vi "Robot Global Data.vi"() -> ()   [LabVIEW 2013]
doc: "This global VI can contain as many global variables as you need. Place a control on the panel, give it a good name. To read or write to it from a VI, drag the icon to the diagram of that VI. You can also drag from the project. Click on the node to change which global you access. You shouldn't have multiple locations writing to a global or it will cause a race-condition."
uses:
  <vilib>/Rock Robotics/WPI/Camera/WPI_CameraImageSize.ctl
  <vilib>/Rock Robotics/WPI/DriverStation/WPI_DriverStationRobotMode2.ctl
  Encoder Values.ctl
  <vilib>/Rock Robotics/WPI/Joystick/WPI_JoystickButtonState.ctl
  Autonomous Commands.ctl
  Shoot Location.ctl
  UDP Dashboard Packet.ctl
  Autonomous Setpoints.ctl
  Auto Shift Settings.ctl
  Shoot Profile.ctl
  Halo Drive.ctl
  Auto Speed Constants.ctl
  Autonomous Center Line Setpoints.ctl
panel:
  out "UDP Packet":T1={"Feed Angle"=20.0, "Neutral Angle"=25.8, "Autonomous Setpoints"={"Shoot Angle 1"=15.4, "Initial Delay"=0.0, "Disc Count 1"=3.0, "Shoot Time 1"=8000.0, "Distance 1"=6.5, "Two Disc Distance 1"=4.0, "Distance 2"=10.5, "Two Disc Distance 2"=6.0, "Distance 3"=-10.0, "Two Disc Distance 3"=0.0, "Shoot Angle 3"=23.0, "Disc Count 3"=5.0, "Shoot Time 3"=15000.0, "Distance 4"=0.0, "Two Disc Distance 4"=0.0, "Low Gear"=TRUE, "Shoot 1 Post Delay"=250.0}, "Auto Shift"={"Enabled"=FALSE, "Upshift Speed"=20.0, "Downshift Speed"=20.0, "Upshift Throttle"=0.6000000000000001, "Turn Power Diff"=0.7, "Motor Limit"=400.0, "Encoder Limit"=100.0}, "Elevator Angle Offset"=0.0, "Potentiometer Angle"={"Pot M"=42.09, "Pot B"=-65.397}, "Shoot Setpoints"={"Vision"={"Pre RPM"=3500.0, "Main RPM"=4000.0, "Angle"=16.4}, "Back Corner"={"Pre RPM"=3500.0, "Main RPM"=4000.0, "Angle"=16.3}, "Front"={"Pre RPM"=3500.0, "Main RPM"=4000.0, "Angle"=23.5}, "Front Corner"={"Pre RPM"=3500.0, "Main RPM"=4000.0, "Angle"=21.8}, "Half Court"={"Pre RPM"=3500.0, "Main RPM"=4000.0, "Angle"=16.4}, "Full Court"={"Pre RPM"=4500.0, "Main RPM"=5000.0, "Angle"=16.0}, "Pyramid"={"Pre RPM"=2800.0, "Main RPM"=3300.0, "Angle"=28.0}}, "Halo Drive"={"Gains"={"Quickturn_Sens_Low"=1.2, "Quickturn_Sens_High"=1.0, "Speedturn_Sens_Low"=1.5, "Speedturn_Sens_High"=1.7}, "QuickTurn Const"=0.25, "Loading Throttle Limit"=0.5}, "Auto Speed Constants"={"Slowing Distance"=0.5, "High Speed"=0.8999999999999999, "Rampup Time"=500.0, "Low Speed"=0.5, "High Speed (Reverse)"=0.8999999999999999}, "Shooting Delays"={"Unjam On"=100.0, "Unjam Off"=100.0, "Flipper On"=300.0, "Flipper Off"=200.0, "Hopper Up"=100.0}, "Left Roller Pwr"=0.8, "Right Roller Pwr"=0.8, "Elevator PID Gains"={"proportional gain (Kc)"=0.2, "integral time (Ti, min)"=0.0, "derivative time (Td, min)"=0.002}, "Elevator PID Output Range"={"output high"=1.0, "output low"=-1.0}, "Elevator Angle Tolerance"=0.1, "Toggle Ears Delay"=500.0, "Toggle Ears Distance"=2.0, "Unjam Servo Angle"=93.0, "Auton Steer PID gains"={"proportional gain (Kc)"=0.007, "integral time (Ti, min)"=0.0, "derivative time (Td, min)"=0.0}, "Auton Steer output range"={"output high"=1.0, "output low"=-1.0}, "Auto Reverse Speed"=0.2, "Auto Stop Throttle"=0.0, "Auto Stop Duration"=0.0, "Spin output range"={"output high"=1.0, "output low"=-1.0}, "Spin PID gains"={"proportional gain (Kc)"=0.4, "integral time (Ti, min)"=0.0, "derivative time (Td, min)"=0.0}, "Auto-Center Line"={"Arc Turn x-axis"=0.0, "Arc Turn y-axis"=0.8999999999999999, "Arc Turn Distance"=-11.0, "Distance 1"=11.0, "Two Disc Distance 1"=0.0, "Distance 2"=-2.0, "Two Disc Distance 2"=0.0, "Spin Angle"=-70.0, "Spin Angle tolerance"=5.0, "Spin y-axis"=0.0, "Spin Distance"=0.0, "Center Line Enabled"=FALSE, "Distance 3"=12.0, "Two Disc Distance 3"=0.0, "Spin Angle 2"=85.0, "Spin Angle tolerance 2"=15.0, "Spin y-axis 2"=0.0, "Spin Distance 2"=0.0, "Shoot Angle 1"=14.6, "Disc Count 1"=3.0, "Shoot Time 1"=8000.0, "Shoot Angle 3"=18.4, "Disc Count 3"=5.0, "Shoot Time 3"=15000.0, "Low Gear"=TRUE}, "Auton Distance PID gains Low Gear"={"proportional gain (Kc)"=0.9999999999999999, "integral time (Ti, min)"=0.007, "derivative time (Td, min)"=0.0}, "Auton Distance output range"={"output high"=0.9, "output low"=-0.9}, "Auton Distance Threshold"=0.25, "Auton Velocity Cutoff"=1.5, "Auton Distance output range Center Line"={"output high"=1.0, "output low"=-1.0}, "Auton Distance PID gains High Gear"={"proportional gain (Kc)"=0.9999999999999999, "integral time (Ti, min)"=0.007, "derivative time (Td, min)"=0.0}} {"Auton Distance PID gains High Gear"."derivative time (Td, min)" format="%.3f"; "Auton Distance PID gains High Gear"."integral time (Ti, min)" format="%.3f"; "Auton Distance PID gains High Gear"."proportional gain (Kc)" format="%.3f"; "Auton Distance PID gains Low Gear"."derivative time (Td, min)" format="%.3f"; "Auton Distance PID gains Low Gear"."integral time (Ti, min)" format="%.3f"; "Auton Distance PID gains Low Gear"."proportional gain (Kc)" format="%.3f"; "Spin PID gains"."derivative time (Td, min)" format="%.3f"; "Spin PID gains"."integral time (Ti, min)" format="%.3f"; "Spin PID gains"."proportional gain (Kc)" format="%.3f"; "Spin output range"."output low" format="%.2f"; "Spin output range"."output high" format="%.2f"; "Auton Steer PID gains"."derivative time (Td, min)" format="%.3f"; "Auton Steer PID gains"."integral time (Ti, min)" format="%.3f"; "Auton Steer PID gains"."proportional gain (Kc)" format="%.3f"}
  in  "Shoot Location":T8
  in  "Auton Commands":T9
  in  "Azimuth Low Gear":bool
  in  "Azimuth Ready":bool
  out "Gryo Angle":dbl
  out "Drive Controls":T10
  in  "Shooter Mode":T11(ring)=enum."Neutral Angle"
  out "Disc Count":dbl
  in  "RPM Min Percentage":dbl
  in  "RPM Max Percentage":dbl
  in  "Bangbang Smooth":dbl
  in  "Target Pre RPM":dbl
  in  "Elevator Target Angle":dbl
  out "IR Sensors":T12
  out "Joysticks":T14
  in  "Drive Limit":bool
  in  "Disc Mode":enum16{"Drive", "Load", "Shoot", "Feed"}(ring)
  in  "Shooter Manual Power":bool
  out "Encoder Values":T15
  in  "Low Gear":bool
  in  "Shooter Active":bool
  in  "Target Main RPM":dbl
  in  "Robot Mode":T16
  in  "LED toggle rate (ms)":u32=20
  in  "image size":T17=enum."320x240"
  in  "Enable Vision":bool
  # "\"Target\" is one of the choices in UDP packet,\nbased on the driver's \"shoot location\""
  # "Low level, controlled by\nShooter Mode in auto loop"
  # "High level, auto controlled state"
  # "Pre RPM"
  # "Main RPM"
  # "Angle"
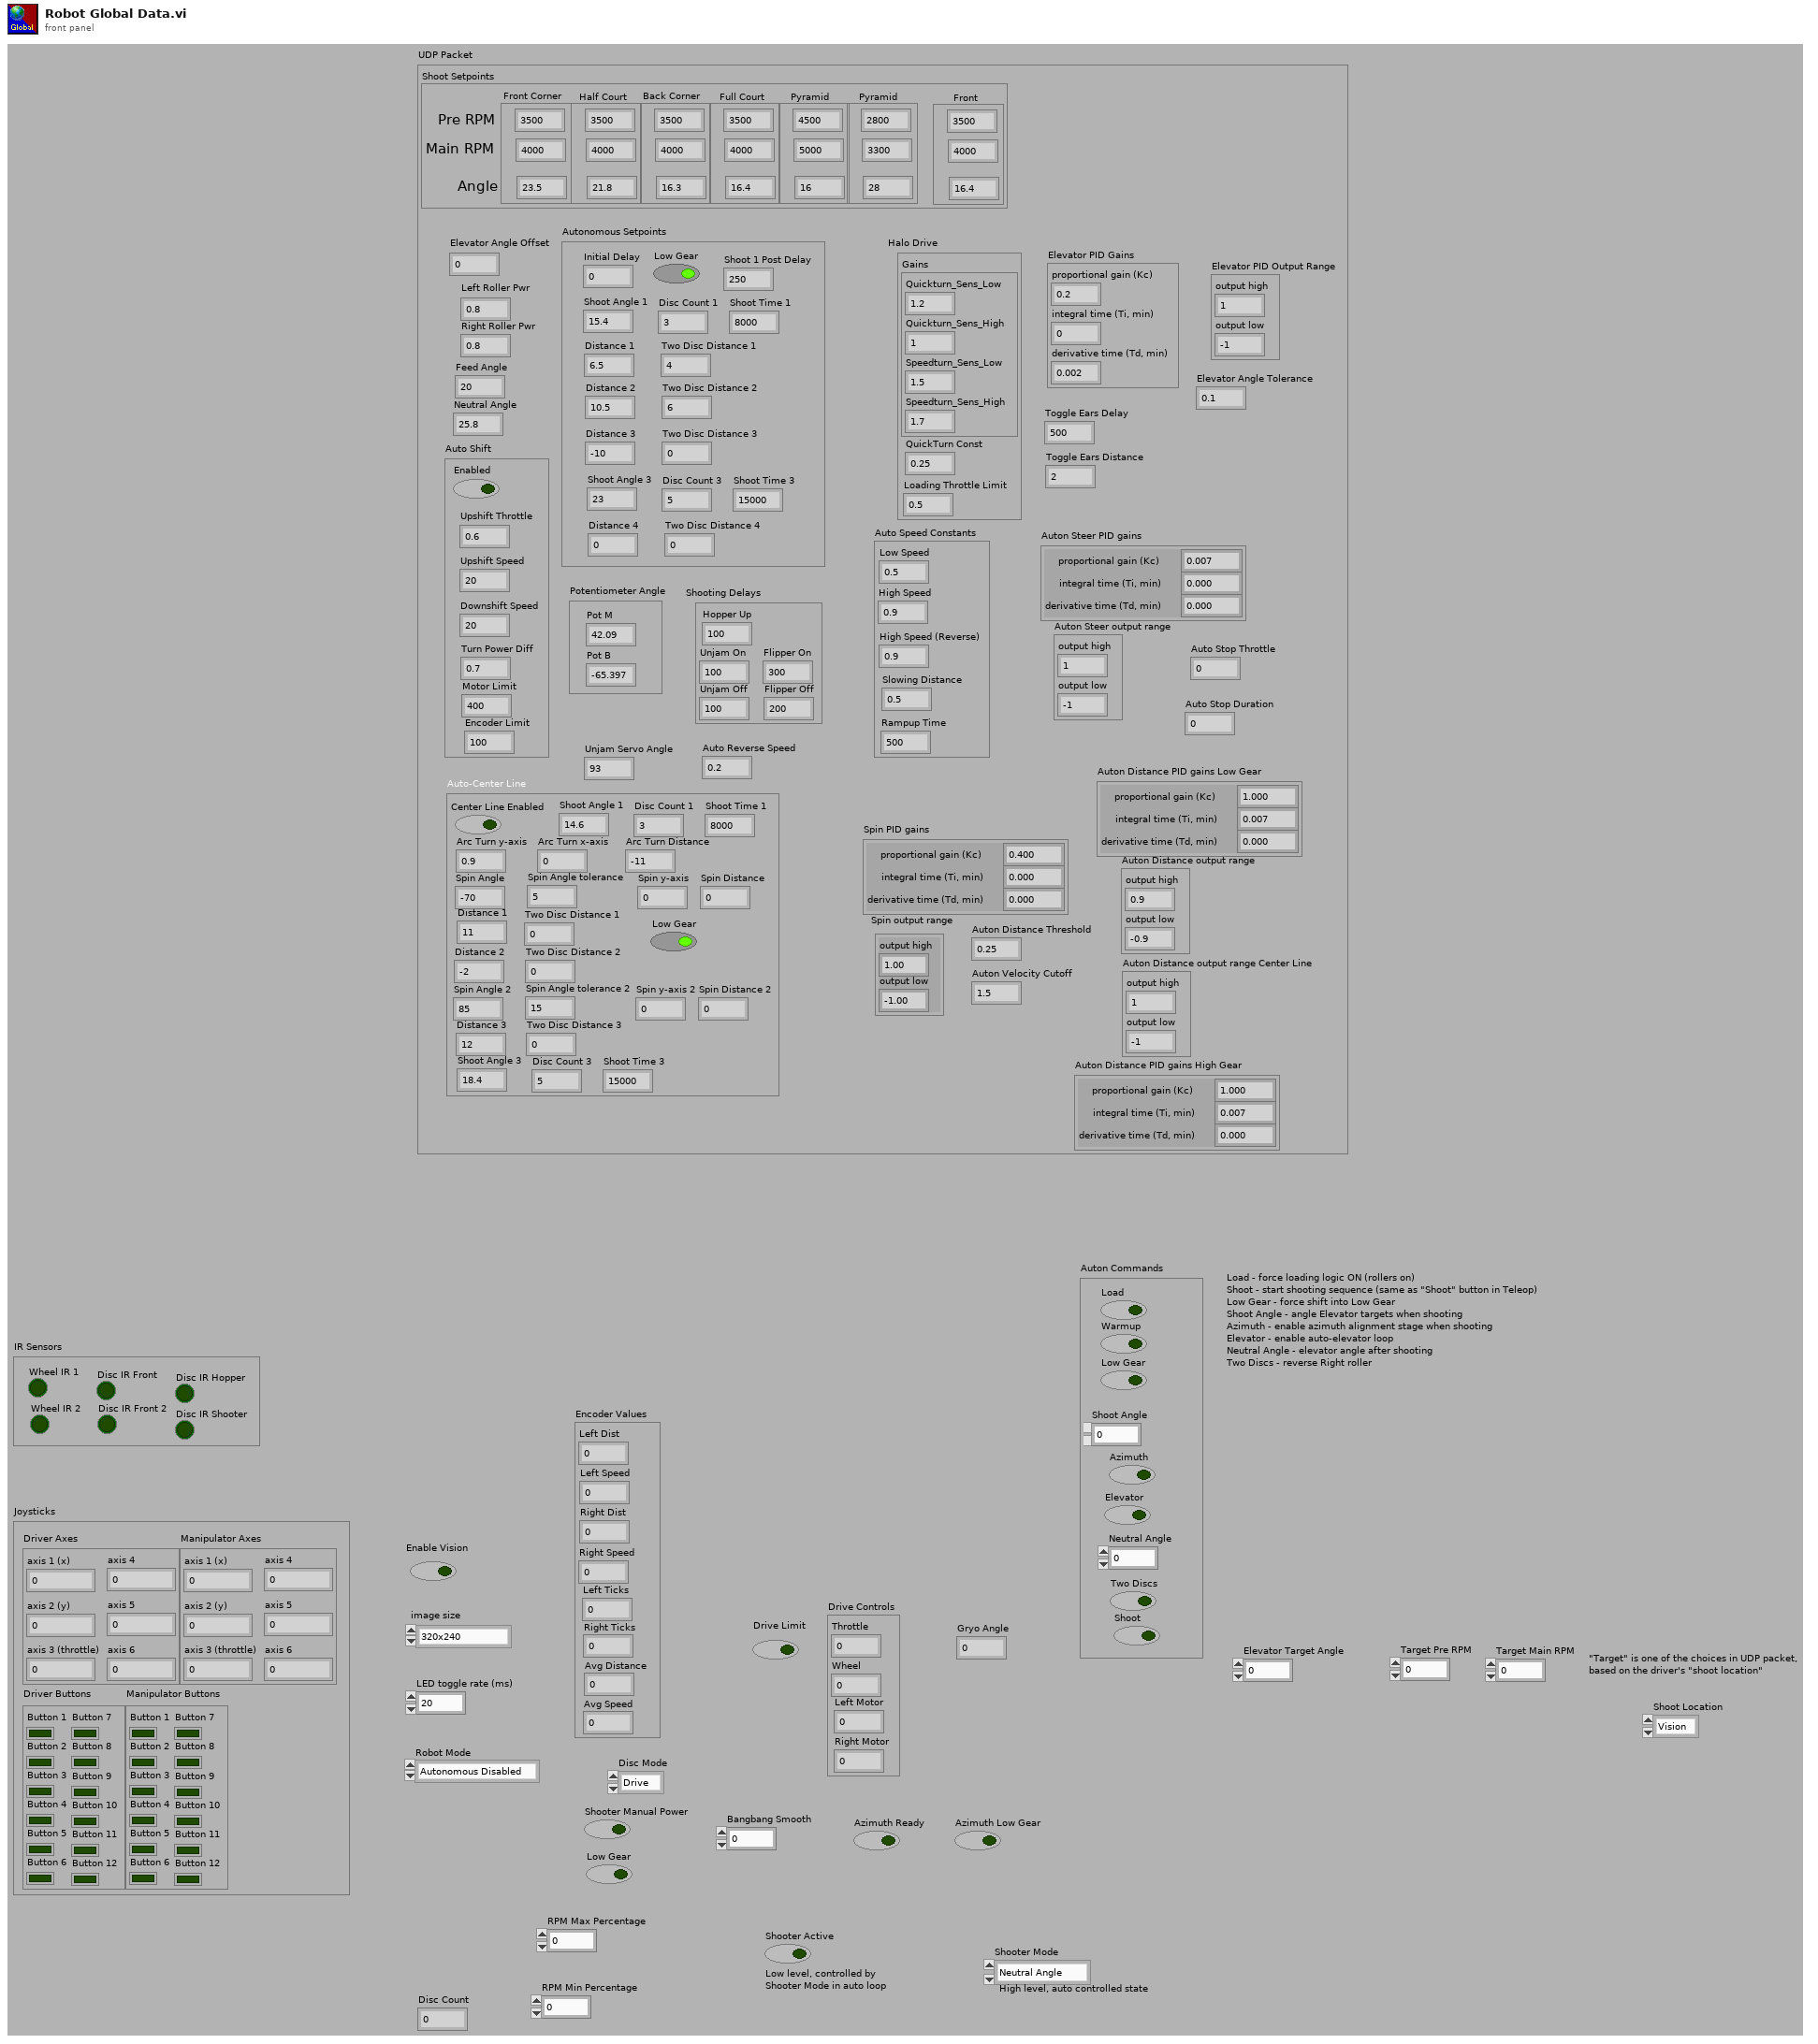
[diagram p1: front panel]
types:
  T1 = typedef "UDP Dashboard Packet.ctl" = cluster{"Feed Angle":dbl, "Neutral Angle":dbl, "Autonomous Setpoints":T2, "Auto Shift":T3, "Elevator Angle Offset":dbl, "Potentiometer Angle":cluster{"Pot M":dbl, "Pot B":dbl}, "Shoot Setpoints":cluster{"Vision":T4, "Back Corner":T4, "Front":T4, "Front Corner":T4, "Half Court":T4, "Full Court":T4, "Pyramid":T4}, "Halo Drive":T5, "Auto Speed Constants":T6, "Shooting Delays":cluster{"Unjam On":dbl, "Unjam Off":dbl, "Flipper On":dbl, "Flipper Off":dbl, "Hopper Up":dbl}, "Left Roller Pwr":dbl, "Right Roller Pwr":dbl, "Elevator PID Gains":cluster{"proportional gain (Kc)":dbl, "integral time (Ti, min)":dbl, "derivative time (Td, min)":dbl}, "Elevator PID Output Range":cluster{"output high":dbl, "output low":dbl}, "Elevator Angle Tolerance":dbl, "Toggle Ears Delay":dbl, "Toggle Ears Distance":dbl, "Unjam Servo Angle":dbl, "Auton Steer PID gains":cluster{"proportional gain (Kc)":dbl, "integral time (Ti, min)":dbl, "derivative time (Td, min)":dbl}, "Auton Steer output range":cluster{"output high":dbl, "output low":dbl}, "Auto Reverse Speed":dbl, "Auto Stop Throttle":dbl, "Auto Stop Duration":dbl, "Spin output range":cluster{"output high":dbl, "output low":dbl}, "Spin PID gains":cluster{"proportional gain (Kc)":dbl, "integral time (Ti, min)":dbl, "derivative time (Td, min)":dbl}, "Auto-Center Line":T7, "Auton Distance PID gains Low Gear":cluster{"proportional gain (Kc)":dbl, "integral time (Ti, min)":dbl, "derivative time (Td, min)":dbl}, "Auton Distance output range":cluster{"output high":dbl, "output low":dbl}, "Auton Distance Threshold":dbl, "Auton Velocity Cutoff":dbl, "Auton Distance output range Center Line":cluster{"output high":dbl, "output low":dbl}, "Auton Distance PID gains High Gear":cluster{"proportional gain (Kc)":dbl, "integral time (Ti, min)":dbl, "derivative time (Td, min)":dbl}}
  T2 = typedef "Autonomous Setpoints.ctl" = cluster{"Shoot Angle 1":dbl, "Initial Delay":dbl, "Disc Count 1":dbl, "Shoot Time 1":dbl, "Distance 1":dbl, "Two Disc Distance 1":dbl, "Distance 2":dbl, "Two Disc Distance 2":dbl, "Distance 3":dbl, "Two Disc Distance 3":dbl, "Shoot Angle 3":dbl, "Disc Count 3":dbl, "Shoot Time 3":dbl, "Distance 4":dbl, "Two Disc Distance 4":dbl, "Low Gear":bool, "Shoot 1 Post Delay":dbl}
  T3 = typedef "Auto Shift Settings.ctl" = cluster{"Enabled":bool, "Upshift Speed":dbl, "Downshift Speed":dbl, "Upshift Throttle":dbl, "Turn Power Diff":dbl, "Motor Limit":dbl, "Encoder Limit":dbl}
  T4 = typedef "Shoot Profile.ctl" = cluster{"Pre RPM":dbl, "Main RPM":dbl, "Angle":dbl}
  T5 = typedef "Halo Drive.ctl" = cluster{"Gains":cluster{"Quickturn_Sens_Low":dbl, "Quickturn_Sens_High":dbl, "Speedturn_Sens_Low":dbl, "Speedturn_Sens_High":dbl}, "QuickTurn Const":dbl, "Loading Throttle Limit":dbl}
  T6 = typedef "Auto Speed Constants.ctl" = cluster{"Slowing Distance":dbl, "High Speed":dbl, "Rampup Time":dbl, "Low Speed":dbl, "High Speed (Reverse)":dbl}
  T7 = typedef "Autonomous Center Line Setpoints.ctl" = cluster{"Arc Turn x-axis":dbl, "Arc Turn y-axis":dbl, "Arc Turn Distance":dbl, "Distance 1":dbl, "Two Disc Distance 1":dbl, "Distance 2":dbl, "Two Disc Distance 2":dbl, "Spin Angle":dbl, "Spin Angle tolerance":dbl, "Spin y-axis":dbl, "Spin Distance":dbl, "Center Line Enabled":bool, "Distance 3":dbl, "Two Disc Distance 3":dbl, "Spin Angle 2":dbl, "Spin Angle tolerance 2":dbl, "Spin y-axis 2":dbl, "Spin Distance 2":dbl, "Shoot Angle 1":dbl, "Disc Count 1":dbl, "Shoot Time 1":dbl, "Shoot Angle 3":dbl, "Disc Count 3":dbl, "Shoot Time 3":dbl, "Low Gear":bool}
  T8 = typedef "Shoot Location.ctl" = enum16{"Vision", "Front", "Front Corner", "Back Corner", "Half Court", "Full Court", "Pyramid"}
  T9 = typedef "Autonomous Commands.ctl" = cluster{"Load":bool, "Warmup":bool, "Low Gear":bool, "Shoot Angle":dbl, "Azimuth":bool, "Elevator":bool, "Neutral Angle":dbl, "Two Discs":bool, "Shoot":bool}
  T10 = cluster{"Throttle":dbl, "Wheel":dbl, "Right Motor":dbl, "Left Motor":dbl}
  T11 = enum16{"Wait", "Adjust Angle", "Warmup Shooter", "Fire", "Feeding", "Neutral Angle"}
  T12 = cluster{"Wheel IR 1":bool, "Wheel IR 2":bool, "Disc IR Front":bool, "Disc IR Front 2":bool, "Disc IR Hopper":bool, "Disc IR Shooter":bool}
  T13 = typedef "WPI_JoystickButtonState.ctl" = cluster{"Button 1":bool, "Button 2":bool, "Button 3":bool, "Button 4":bool, "Button 5":bool, "Button 6":bool, "Button 7":bool, "Button 8":bool, "Button 9":bool, "Button 10":bool, "Button 11":bool, "Button 12":bool}
  T14 = cluster{"Driver Axes":cluster{"axis 1 (x)":dbl, "axis 2 (y)":dbl, "axis 3 (throttle)":dbl, "axis 4":dbl, "axis 5":dbl, "axis 6":dbl}, "Driver Buttons":T13, "Manipulator Axes":cluster{"axis 1 (x)":dbl, "axis 2 (y)":dbl, "axis 3 (throttle)":dbl, "axis 4":dbl, "axis 5":dbl, "axis 6":dbl}, "Manipulator Buttons":T13}
  T15 = typedef "Encoder Values.ctl" = cluster{"Left Dist":dbl, "Left Speed":dbl, "Right Dist":dbl, "Right Speed":dbl, "Left Ticks":dbl, "Right Ticks":dbl, "Avg Distance":dbl, "Avg Speed":dbl}
  T16 = typedef "WPI_DriverStationRobotMode2.ctl" = enum16{"Autonomous Disabled", "Autonomous Enabled", "Teleop Disabled", "Teleop Enabled", "Timeout", "Finish", "Test Disabled", "Test Enabled"}
  T17 = typedef "WPI_CameraImageSize.ctl" = enum16{"640x480", "320x240", "160x120"}
diagram:
